vi "get_laser_energy.vi"(8 "Index":i32=-8900 min=-20000 max=20000 step=1, 9 "HWP angle":dbl caption="HWP angle [degree]" format="%#_13g", 11 "Astrella Power":dbl[](array[numeric]) caption="Astrella Power [mW]") -> (0 "Attenuated Power":dbl caption="Attenuated Power [mW]", 1 "HCF output power":dbl caption="HCF output power [mW]", 3 "FF input energy":dbl caption="FF input energy [uJ]")   [LabVIEW 2020]
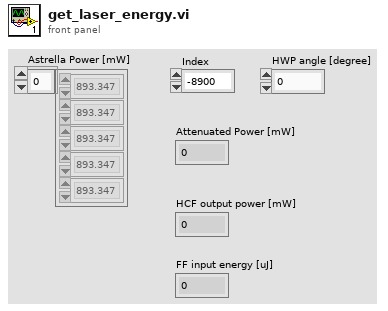
[diagram p1: front panel]
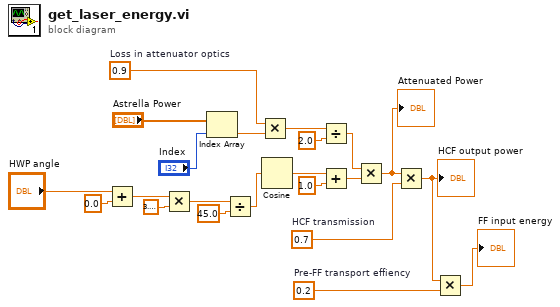
[diagram p0: block diagram]
diagram:
  w6 = 0.2  # Pre-FF transport effiency
  w8 = 0.7  # HCF transmission
  w16 = 0.9  # Loss in attenuator optics
  n1 = Add(x="HWP angle", y=0.0) -> (x+y=w15:dbl)
  n2 = Multiply(x=w15, y=3.141592653589793) -> (x*y=w22:dbl)
  n3 = Index Array(array="Astrella Power", index="Index") -> (element=w11:dbl)
  n4 = Divide(x=w22, y=45.0) -> (x/y=w20:dbl)
  n5 = Multiply(x=w16, y=w11) -> (x*y=w1:dbl)
  n6 = Cosine(x=w20) -> (cos(x)=w19:dbl)
  n7 = Divide(x=w1, y=2.0) -> (x/y=w3:dbl)
  n8 = Add(x=w19, y=1.0) -> (x+y=w18:dbl)
  n9 = Multiply(x=w3, y=w18) -> (x*y=w4:dbl)
  "Attenuated Power" <- w4
  n10 = Multiply(x=w4, y=w8) -> (x*y=w7:dbl)
  "HCF output power" <- w7
  n11 = Multiply(x=w7, y=w6) -> (x*y=→"FF input energy":dbl)
